vi "Write Single Coil.vi"(8 "error in (no error)":errorcluster, 9 "coil value":bool, 10 "address":u16, 11 "Modbus master in":refnum<class "Network Master.lvclass">) -> (0 "error out":errorcluster, 3 "Modbus master out":refnum<class "Network Master.lvclass">)   [LabVIEW 2021, in "Network Master.lvclass"]
doc: "Writes a value to a single coil."
uses:
  Network Master.lvclass
  Modbus Data Unit/Modbus Data Unit.lvclass/Modbus Data Unit.ctl
  Network Master.lvclass/Network Master.ctl
  Modbus Data Unit/Construct PDU.vi
  Data Model/Error Generator.vi
  Master Function Definition/Function code mismatch error.vi
  Modbus Data Unit/Deconstruct PDU.vi
  Modbus Data Unit/Modbus Data Unit.lvclass
  Transmission Data Unit/Transmission Data Unit.lvclass
  Master Function Definition/Master Function Definition.lvclass
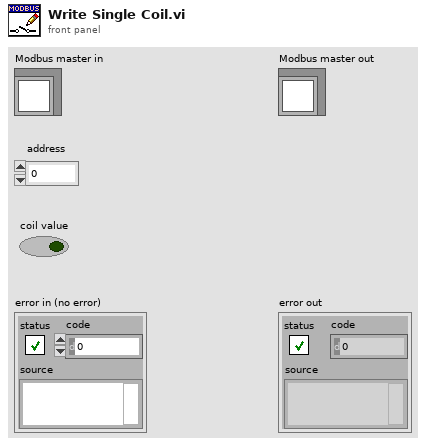
[diagram p1: front panel]
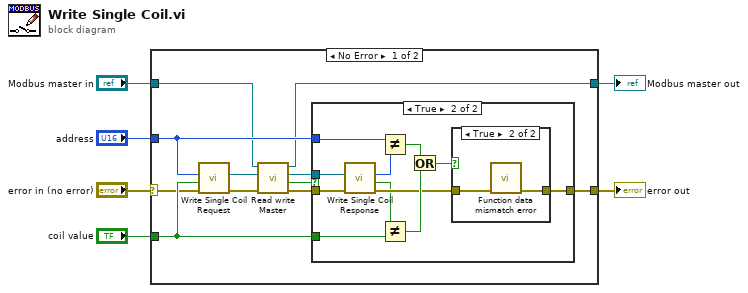
[diagram p0: block diagram]
diagram:
  n1 = case shown="No Error" "error in (no error)" {
    selector: "error in (no error)" -> [w7 w34]
    tunnel: "Modbus master in" -> [w8 w33]
    tunnel: [w16 w34] -> w3
    tunnel: [w9 w33] -> w2
    tunnel: "address" -> [w13 _]
    tunnel: "coil value" -> [w15 _]
    frame No Error {
      n2 = call "Write Single Coil Request.vi"("error in"=w7, "Coil Value"=w15, "Starting Address"=w13) -> ("error out"=w17:errorcluster, "modbus data unit out"=w10:refnum<class "Modbus Data Unit.lvclass">)  [unwired: 7 in]
      n3 = call "Read write Master.vi"("error in (no error)"=w17, "Modbus data unit in"=w10, "Modbus master in"=w8) -> ("error out"=w14:errorcluster, "PDU valid?"=w12:bool, "Modbus data unit out"=w11:refnum<class "Modbus Data Unit.lvclass">, "Modbus master out"=w9:refnum<class "Network Master.lvclass">)  [unwired: 5 in]
      n4 = case shown="True" w12 {
        tunnel: [w18 w28] -> w16
        tunnel: w15 -> [_ w20]
        tunnel: w14 -> [w18 w24]
        tunnel: w11 -> [_ w23]
        tunnel: w13 -> [_ w21]
        frame False {
        }
        frame True {
          n5 = call "Write Single Coil Response.vi"("error in"=w24, "modbus data unit in"=w23) -> ("error out"=w22:errorcluster, "Coil Value"=w19:bool, "Address"=w25:u16)  [unwired: 7 in]
          n6 = Not Equal?(x=w21, y=w25) -> (x != y?=w27:bool)
          n7 = Not Equal?(x=w19, y=w20) -> (x != y?=w26:bool)
          n8 = Or(x=w27, y=w26) -> (x .or. y?=w29:bool)
          n9 = case shown="True" w29 {
            tunnel: [w30 w32] -> w28
            tunnel: w22 -> [w30 w31]
            frame False {
            }
            frame True {
              n10 = call "Function data mismatch error.vi"("error in (no error)"=w31) -> ("error out"=w32:errorcluster)  [unwired: 10 in]
            }
          }
        }
      }
    }
    frame Error {
    }
  }
  "error out" <- w3
  "Modbus master out" <- w2
